vi "Set All Names and Values.vi"(6 "Cluster Name":string, 8 "error in":errorcluster, 9 "values":variant[](array[variant]), 10 "Element Names":string[](array[string]), 11 "Cluster in":variant) -> (0 "error out":errorcluster, 3 "Cluster out":variant)   [LabVIEW 2017, in "Variant Data Manipulation.lvlib"]
doc: "Returns an array of all of the keys and an array of their corresponding values. Elements are correlated by index, so the key at a given index corresponds to the value at the same index."
uses:
  Variant Data Manipulation.lvlib
  <vilib>/Utility/Data Type/NI_Data Type.lvlib
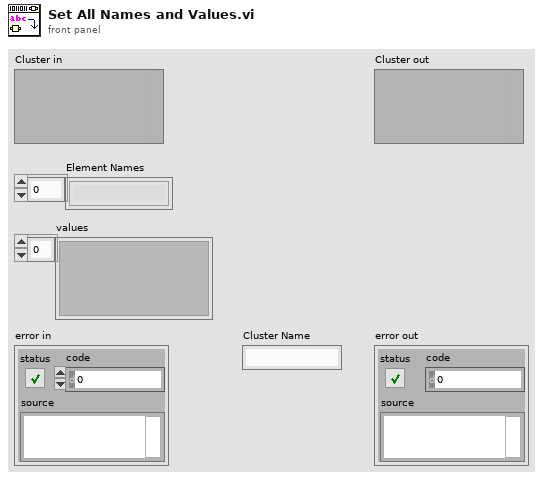
[diagram p1: front panel]
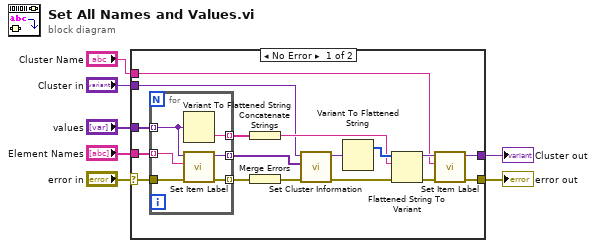
[diagram p0: block diagram]
diagram:
  n1 = case shown="No Error" "error in" {
    selector: "error in" -> [w13 w31]
    tunnel: "Cluster in" -> [w10 w32]
    tunnel: "values" -> [w18 _]
    tunnel: [w15 w32] -> w5
    tunnel: [w14 w31] -> w3
    tunnel: "Element Names" -> [w19 _]
    tunnel: "Cluster Name" -> [w8 _]
    frame No Error {
      n2 = for {
        tunnel: w18 -> [w27] mode=indexing
        tunnel: [w30] -> w24 mode=indexing
        tunnel: w19 -> [w29] mode=indexing
        tunnel: [w28] -> w17 mode=indexing
        tunnel: w13 -> [w26]
        tunnel: [w25] -> w12 mode=indexing
        n3 = Variant To Flattened String(Variant=w27) -> (data string=w30:string)  [unwired: 1 out]
        n4 = call "Set Item Label.vi"("error in (no error)"=w26, "Name"=w29, "Variant in"=w27) -> ("error out"=w25:errorcluster, "Variant out"=w28:variant)  [unwired: 7 in]
      }
      n5 = Concatenate Strings(w24) -> (w21:string)
      n6 = Merge Errors(w12) -> (w11:errorcluster)
      n7 = call <vilib>:"Set Cluster Information.vi"("error in (no error)"=w11, "Cluster Elements"=w17, "Variant in"=w10) -> ("error out"=w20:errorcluster, "Variant out"=w23:variant)  [unwired: 7 in]
      n8 = Variant To Flattened String(Variant=w23) -> (1:w22:i16[])  [unwired: 1 out]
      n9 = Flattened String To Variant(4:w20, 6:w21, 7:w22) -> (0:w9:errorcluster, 3:w16:variant)
      n10 = call "Set Item Label.vi"("error in (no error)"=w9, "Name"=w8, "Variant in"=w16) -> ("error out"=w14:errorcluster, "Variant out"=w15:variant)  [unwired: 7 in]
    }
    frame Error {
    }
  }
  "error out" <- w3
  "Cluster out" <- w5
